vi "Get FPGA Time.vi"(8 "error in":errorcluster, 11 "Session In":refnum<k20>) -> (0 "error out":errorcluster, 2 "Time Stamp":timestamp, 3 "Session Out":refnum<k20>)   [LabVIEW 2016]
uses:
  <vilib>/Utility/error.llb/Error Cluster From Error Code.vi
  <vilib>/rvi/errors/niLvFpgaAdjustHostInterfaceError.vi
  <vilib>/rvi/interface/nirviReadWriteControl/nirviReadWriteControl.xnode
  NiFpgaLv.dll
  <vilib>/rvi/interface/Simulation/niFpgaSimulationCallBeginRW.vi
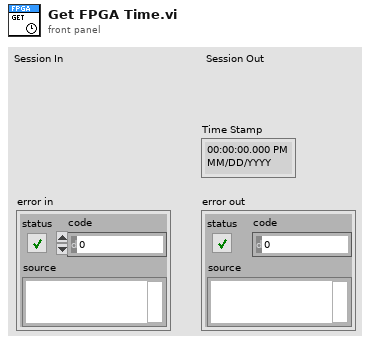
[diagram p1: front panel]
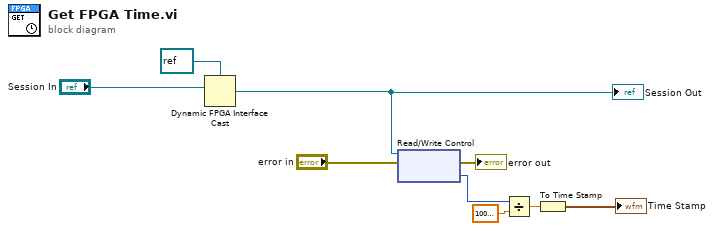
[diagram p0: block diagram]
diagram:
  n1 = Dynamic FPGA Interface Cast(Session In=refnum<k20> refnum ("Type"), Type="Session In") -> (Session Out=w2:refnum<k20>)
  "Session Out" <- w2
  n2 = xnode "Read/Write Control"("FPGA VI Reference In"=w2, "error in"="error in") -> ("error out"=→"error out":errorcluster, "Time-ns"=w6:u64)  [unwired: 1 out]
  n3 = Divide(x=w6, y=1000000000.0) -> (x/y=w8:dbl)
  n4 = To Time Stamp(1:w8) -> (0:→"Time Stamp":timestamp)
